vi "WriteSuccessFile.vi"(8 "error in (no error)":errorcluster, 9 "Generated files":T1[](array[typedef]), 11 "SolutionBuilder in":refnum<class "SolutionBuilder.lvclass">) -> (0 "error out":errorcluster, 3 "SolutionBuilder out":refnum<class "SolutionBuilder.lvclass">)   [LabVIEW 2019, in "SolutionBuilder.lvlib" / "SolutionBuilder.lvclass"]
uses:
  SolutionBuilder.lvclass
  BuildManager/GeneratedFile.ctl
  BuildManager/BuildManager.lvclass
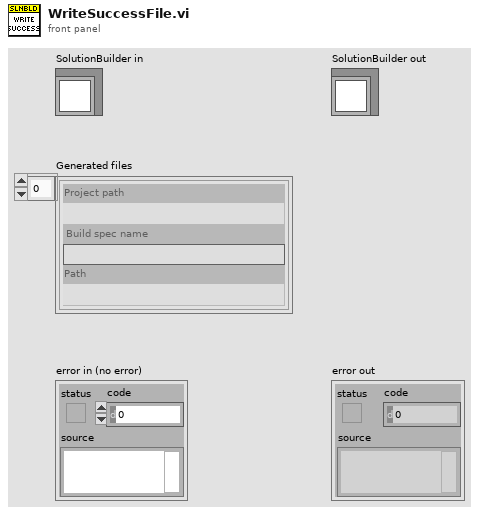
[diagram p1: front panel]
types:
  T1 = typedef "SolutionBuilder.lvlib/BuildManager.lvclass/GeneratedFile.ctl" = cluster{"Project path":path, "Build spec name":string, "Path":path}
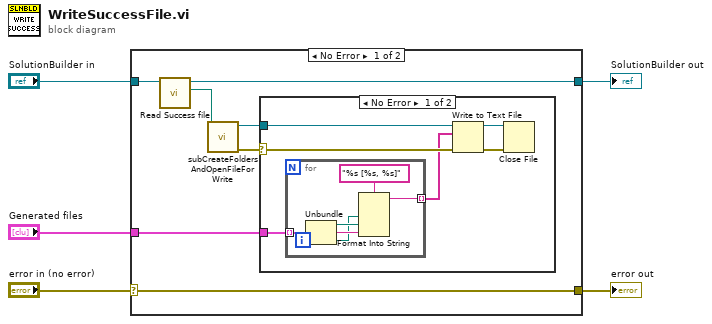
[diagram p0: block diagram]
diagram:
  n1 = case shown="No Error" "error in (no error)" {
    selector: "error in (no error)" -> [w12 w26]
    tunnel: [w12 w26] -> w4
    tunnel: [w11 w25] -> w2
    tunnel: "SolutionBuilder in" -> [w10 w25]
    tunnel: "Generated files" -> [w6 _]
    frame No Error {
      n2 = call-dynamic "Read Success file.vi"("SolutionBuilder in"=w10) -> ("Success file"=w9:path, "SolutionBuilder out"=w11:refnum<class "SolutionBuilder.lvclass">)  [unwired: 9 in]
      n3 = call "subCreateFoldersAndOpenFileForWrite.vi"("File path"=w9) -> ("error out"=w8:errorcluster, "File ref"=w7:refnum<file>)  [unwired: 9 in]
      n4 = case shown="No Error" w8 {
        selector: w8 -> [w17 _]
        tunnel: w7 -> [w18 _]
        tunnel: w6 -> [w16 _]
        frame No Error {
          n5 = for {
            tunnel: w16 -> [w24] mode=indexing
            tunnel: [w19] -> w15 mode=indexing
            n6 = Unbundle(w24) -> ("Project path"=w23:path, "Build spec name"=w22:string, "Path"=w20:path)
            n7 = Format Into String(format string="%s [%s, %s]", w20, w23, w22) -> (resulting string=w19:string)  [unwired: 2 in, 1 out]
          }
          n8 = Write to Text File(file (use dialog)=w18, text=w15, error in=w17) -> (refnum out=w14:refnum<file>, error out=w13:errorcluster)  [unwired: 1 in, 1 out]
          n9 = Close File(refnum=w14, error in=w13) -> ()  [unwired: 2 out]
        }
        frame Error {
        }
      }
    }
    frame Error {
    }
  }
  "error out" <- w4
  "SolutionBuilder out" <- w2
